vi "capt_data_with_visa_rsc.vi"(7 "delay before read (ms)":u32=10, 8 "error in (no error)":errorcluster, 9 "sens_type_arry":T2=[0, 0, 0, 0, 0, 0, 0, 0] items=["SHTC3", "SHT3X", "D6T_1A", "HTS221", "AHT20", "ADT7410"], 10 "wr_buffr":string="\b", 11 "VISA Refnum in":refnum<visa-resource-name>="COM4") -> (0 "error out":errorcluster, 1 "bytes read":u32, 2 "Response":string, 3 "VISA Refnum out":refnum<visa-resource-name>, 4 "equal":bool)   [LabVIEW 2013]
uses:
  sens_type_arry_cntrl.ctl
  sens_type.ctl
  prog_files_all/ni/labview/examples/Instrument IO/Serial/support/Serial - Settings.ctl
  <vilib>/Instr/_visa.llb/VISA Configure Serial Port (Instr).vi
panel:
  in  "wait_after_init":u32
  in  "Serial Settings":T1={"baud rate"=19200, "data bits"=8, "parity"=enum."None", "stop bits"=10, "flow control"=0} {"flow control" items=["None"=0, "XON/XOFF"=1, "RTS/CTS"=2, "DTR/DSR"=4]; "stop bits" items=["1.0"=10, "1.5"=15, "2.0"=20]; "data bits" min=5 max=8 step=1; "baud rate" items=["75"=75, "110"=110, "134"=134, "150"=150, "300"=300, "600"=600, "1200"=1200, "1800"=1800, "2400"=2400, "4800"=4800, "7200"=7200, "9600"=9600, "14400"=14400, "19200"=19200, "28800"=28800, "38400"=38400, "56000"=56000, "57600"=57600, "115200"=115200, "128000"=128000, "230400"=230400]}
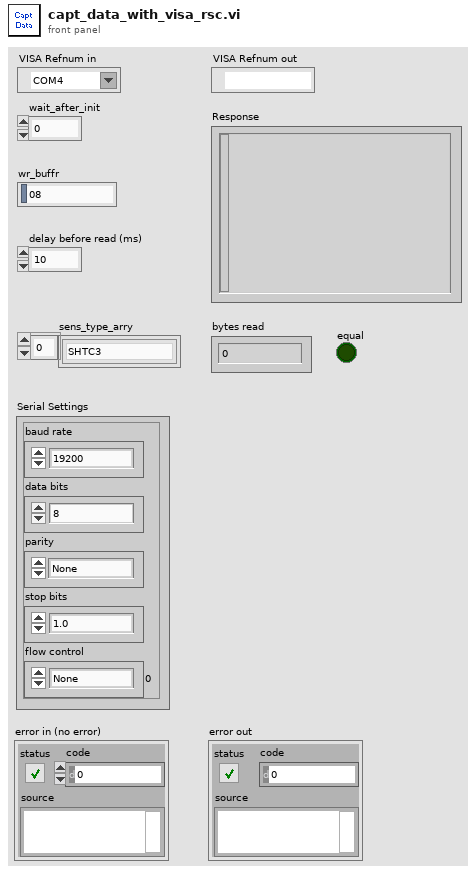
[diagram p1: front panel]
types:
  T1 = typedef "Serial - Settings.ctl" = cluster{"baud rate":u32, "data bits":u16, "parity":enum16{"None", "Odd", "Even", "Mark", "Space"}, "stop bits":u16, "flow control":u16}
  T2 = typedef "sens_type_arry_cntrl.ctl" = T3[]
  T3 = typedef "sens_type.ctl" = u8
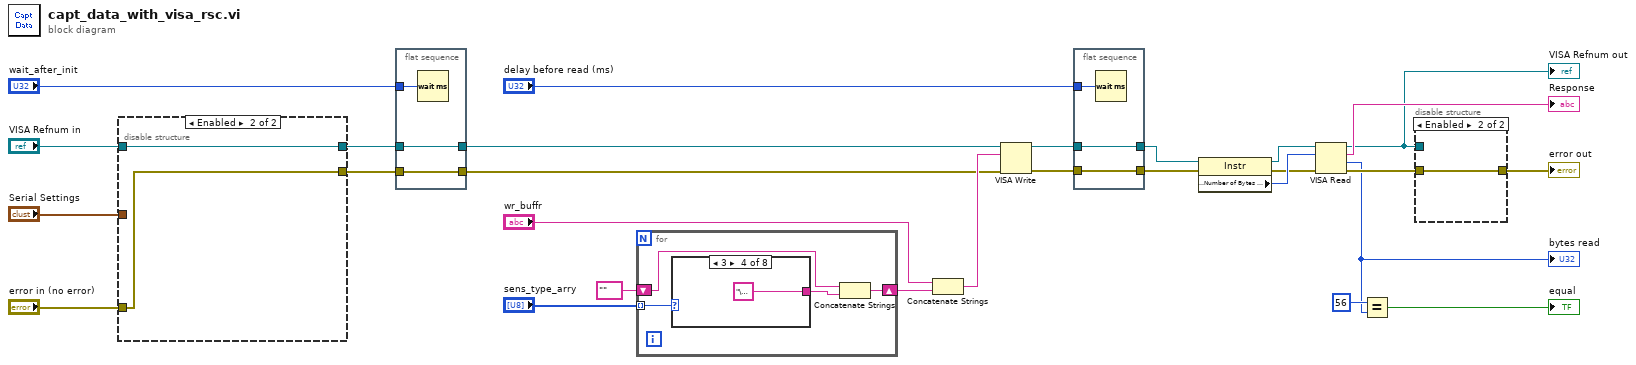
[diagram p0: block diagram]
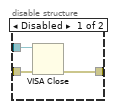
[diagram p2: hidden frame]
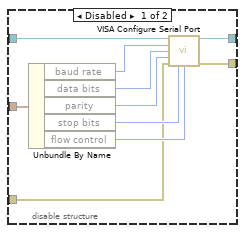
[diagram p3: hidden frame]
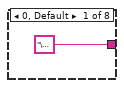
[diagram p4: hidden frame]
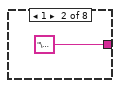
[diagram p5: hidden frame]
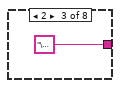
[diagram p6: hidden frame]
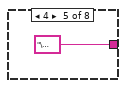
[diagram p7: hidden frame]
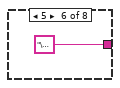
[diagram p8: hidden frame]
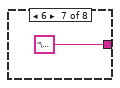
[diagram p9: hidden frame]
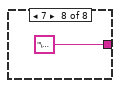
[diagram p10: hidden frame]
diagram:
  n1 = disable-structure shown="Enabled" {
    disable-tunnel: "Serial Settings" -> [w38 _]
    disable-tunnel: "VISA Refnum in" -> [w34 w40]
    disable-tunnel: "error in (no error)" -> [w31 w39]
    disable-tunnel: [w30 w40] -> w5
    disable-tunnel: [w29 w39] -> w3
    frame Disabled {
      n2 = Unbundle By Name(w38) -> ("baud rate"=w33:u32, "data bits"=w32:u16, "parity"=w37:enum16{"None", "Odd", "Even", "Mark", "Space"}, "stop bits"=w36:u16, "flow control"=w35:u16)
      n3 = call-poly "VISA Configure Serial Port"("VISA resource name"=w34, "baud rate (9600)"=w33, "data bits (8)"=w32, "parity (0:none)"=w37, "error in (no error)"=w31, "stop bits (10: 1 bit)"=w36, "flow control (0:none)"=w35) -> ("VISA resource name out"=w30:refnum<visa-resource-name>, "error out"=w29:errorcluster)  [unwired: 2 in, 5 out]
    }
    frame Enabled {
    }
  }
  n4 = flat-sequence {
    tunnel: "wait_after_init" -> [w43]
    tunnel: w5 -> [w42]
    tunnel: [w42] -> w4
    tunnel: w3 -> [w41]
    tunnel: [w41] -> w2
    frame #0 {
      n5 = Wait (ms)(milliseconds to wait=w43) -> ()  [unwired: 1 out]
    }
  }
  n6 = for {
    tunnel: "sens_type_arry" -> [w46] mode=indexing
    shift-right: [w45] -> w25
    shift-left: "" -> [w47]
    n7 = case shown="3" w46 {
      tunnel: ["\u0000" "\u0001" "\u0002" "\u0003" "\u0004" "\u0005" "\u0006" "\u0007"] -> w44
      frame 0, Default {
      }
      frame 1 {
      }
      frame 2 {
      }
      frame 3 {
      }
      frame 4 {
      }
      frame 5 {
      }
      frame 6 {
      }
      frame 7 {
      }
    }
    n8 = Concatenate Strings(w47, w44) -> (w45:string)
  }
  n9 = Concatenate Strings("wr_buffr", w25) -> (w28:string)
  n10 = VISA Write(VISA resource name=w4, write buffer=w28, error in (no error)=w2) -> (VISA resource name out=w17:refnum<visa-resource-name>, error out=w15:errorcluster)  [unwired: 1 out]
  n11 = flat-sequence {
    tunnel: w15 -> [w58]
    tunnel: [w58] -> w16
    tunnel: w17 -> [w57]
    tunnel: [w57] -> w18
    tunnel: "delay before read (ms)" -> [w56]
    frame #0 {
      n12 = Wait (ms)(milliseconds to wait=w56) -> ()  [unwired: 1 out]
    }
  }
  n13 = property class="Instr"(reference=w18, error in=w16) -> (reference out=w19:refnum<visa-resource-name>, error out=w20:errorcluster, "Serial Settings:Number of Bytes at Serial Port"=w21:u32)
  n14 = VISA Read(VISA resource name=w19, byte count=w21, error in (no error)=w20) -> (VISA resource name out=w10:refnum<visa-resource-name>, read buffer=→"Response":string, return count=w7:u32, error out=w11:errorcluster)
  "bytes read" <- w7
  "VISA Refnum out" <- w10
  n15 = Equal?(x=u32 56, y=w7) -> (x = y?=→"equal":bool)
  n16 = disable-structure shown="Enabled" {
    disable-tunnel: w11 -> [w61 w62]
    disable-tunnel: w10 -> [w60 _]
    disable-tunnel: [w59 w62] -> w9
    frame Disabled {
      n17 = VISA Close(VISA resource name=w60, error in (no error)=w61) -> (error out=w59:errorcluster)
    }
    frame Enabled {
    }
  }
  "error out" <- w9
